vi "initialization.vi"(9 "软件版本":refnum<vi>, 10 "updateconfiguration":refnum<vi>) -> ()   [LabVIEW 2016, in "数据传输系统.lvlib"]
uses:
  <vilib>/Utility/config.llb/Read Key (String).vi
  <vilib>/Utility/config.llb/NI_LVConfig.lvlib
panel:
  in  "参数数值":T1={"CODMn"=TRUE, "CODCr"=TRUE, "DO"=TRUE, "铜"=TRUE, "PH"=TRUE, "氨氮"=TRUE, "比电导率"=TRUE, "水温"=TRUE, "COD"=TRUE, "浊度"=TRUE, "总氮"=TRUE, "总磷"=TRUE, "叶绿素a"=TRUE, "藻密度"=TRUE, "水位"=TRUE, "流速"=TRUE, "瞬时流量"=TRUE, "累积流量"=TRUE, "亚硝氮"=TRUE, "硫化物"=TRUE, "ORP"=TRUE, "铅"=TRUE, "镉"=TRUE, "锌"=TRUE, "镍"=TRUE, "锰"=TRUE, "汞"=TRUE, "气温"=TRUE, "气压"=TRUE, "风速"=TRUE, "风向"=TRUE, "盐度"=TRUE, "磷酸盐"=TRUE, "硝氮"=TRUE, "氟化物"=TRUE, "挥发酚"=TRUE, "氯化物"=TRUE}
  out "配置表格":string[][](table)
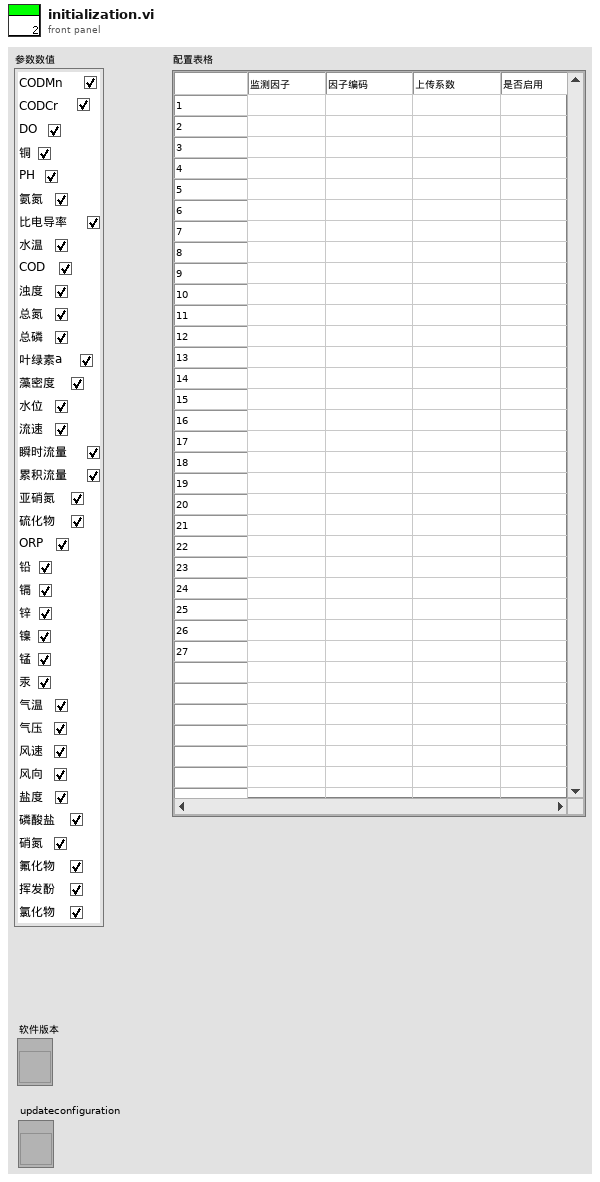
[diagram p1: front panel]
types:
  T1 = cluster{"CODMn":bool, "CODCr":bool, "DO":bool, "铜":bool, "PH":bool, "氨氮":bool, "比电导率":bool, "水温":bool, "COD":bool, "浊度":bool, "总氮":bool, "总磷":bool, "叶绿素a":bool, "藻密度":bool, "水位":bool, "流速":bool, "瞬时流量":bool, "累积流量":bool, "亚硝氮":bool, "硫化物":bool, "ORP":bool, "铅":bool, "镉":bool, "锌":bool, "镍":bool, "锰":bool, "汞":bool, "气温":bool, "气压":bool, "风速":bool, "风向":bool, "盐度":bool, "磷酸盐":bool, "硝氮":bool, "氟化物":bool, "挥发酚":bool, "氯化物":bool}
  T2 = cluster{"setini":string, "sysini":string, "hechaini":string, "actualwrite":string, "actualread":string, "datasent":string, "反控命令信息队列":string, "反控与仪器交互":string}
  T3 = cluster{"主机":string, "用户":string, "密码":string, "远程路径":string, "下载文件名":string, "软件版本":string}
  T4 = cluster{"CODMn":string, "CODCr":string, "DO":string, "铜":string, "PH":string, "氨氮":string, "比电导率":string, "水温":string, "COD":string, "浊度":string, "总氮":string, "总磷":string, "叶绿素a":string, "藻密度":string, "水位":string, "流速":string, "瞬时流量":string, "累积流量":string, "亚硝酸盐":string, "硫化物":string, "ORP":string, "铅":string, "镉":string, "锌":string, "镍":string, "锰":string, "汞":string, "气温":string, "气压":string, "风速":string, "风向":string, "盐度":string, "磷酸盐":string, "硝氮":string, "氟化物":string, "挥发酚":string, "氯化物":string}
  T5 = typedef "NI_LVConfig.lvlib/Config Data RefNum.ctl" = refnum<k1>
  T6 = cluster{"[0]":string, "[1]":string, "[2]":string, "[3]":string, "[4]":string, "[5]":string, "[6]":string, "[7]":string, "[8]":string, "[9]":string, "[10]":string, "[11]":string, "[12]":string, "[13]":string, "[14]":string, "[15]":string, "[16]":string, "[17]":string, "[18]":string, "[19]":string, "[20]":string, "[21]":string, "[22]":string, "[23]":string, "[24]":string, "[25]":string, "[26]":string, "[27]":string, "[28]":string, "[29]":string, "[30]":string, "[31]":string, "[32]":string, "[33]":string, "[34]":string, "[35]":string, "[36]":string}
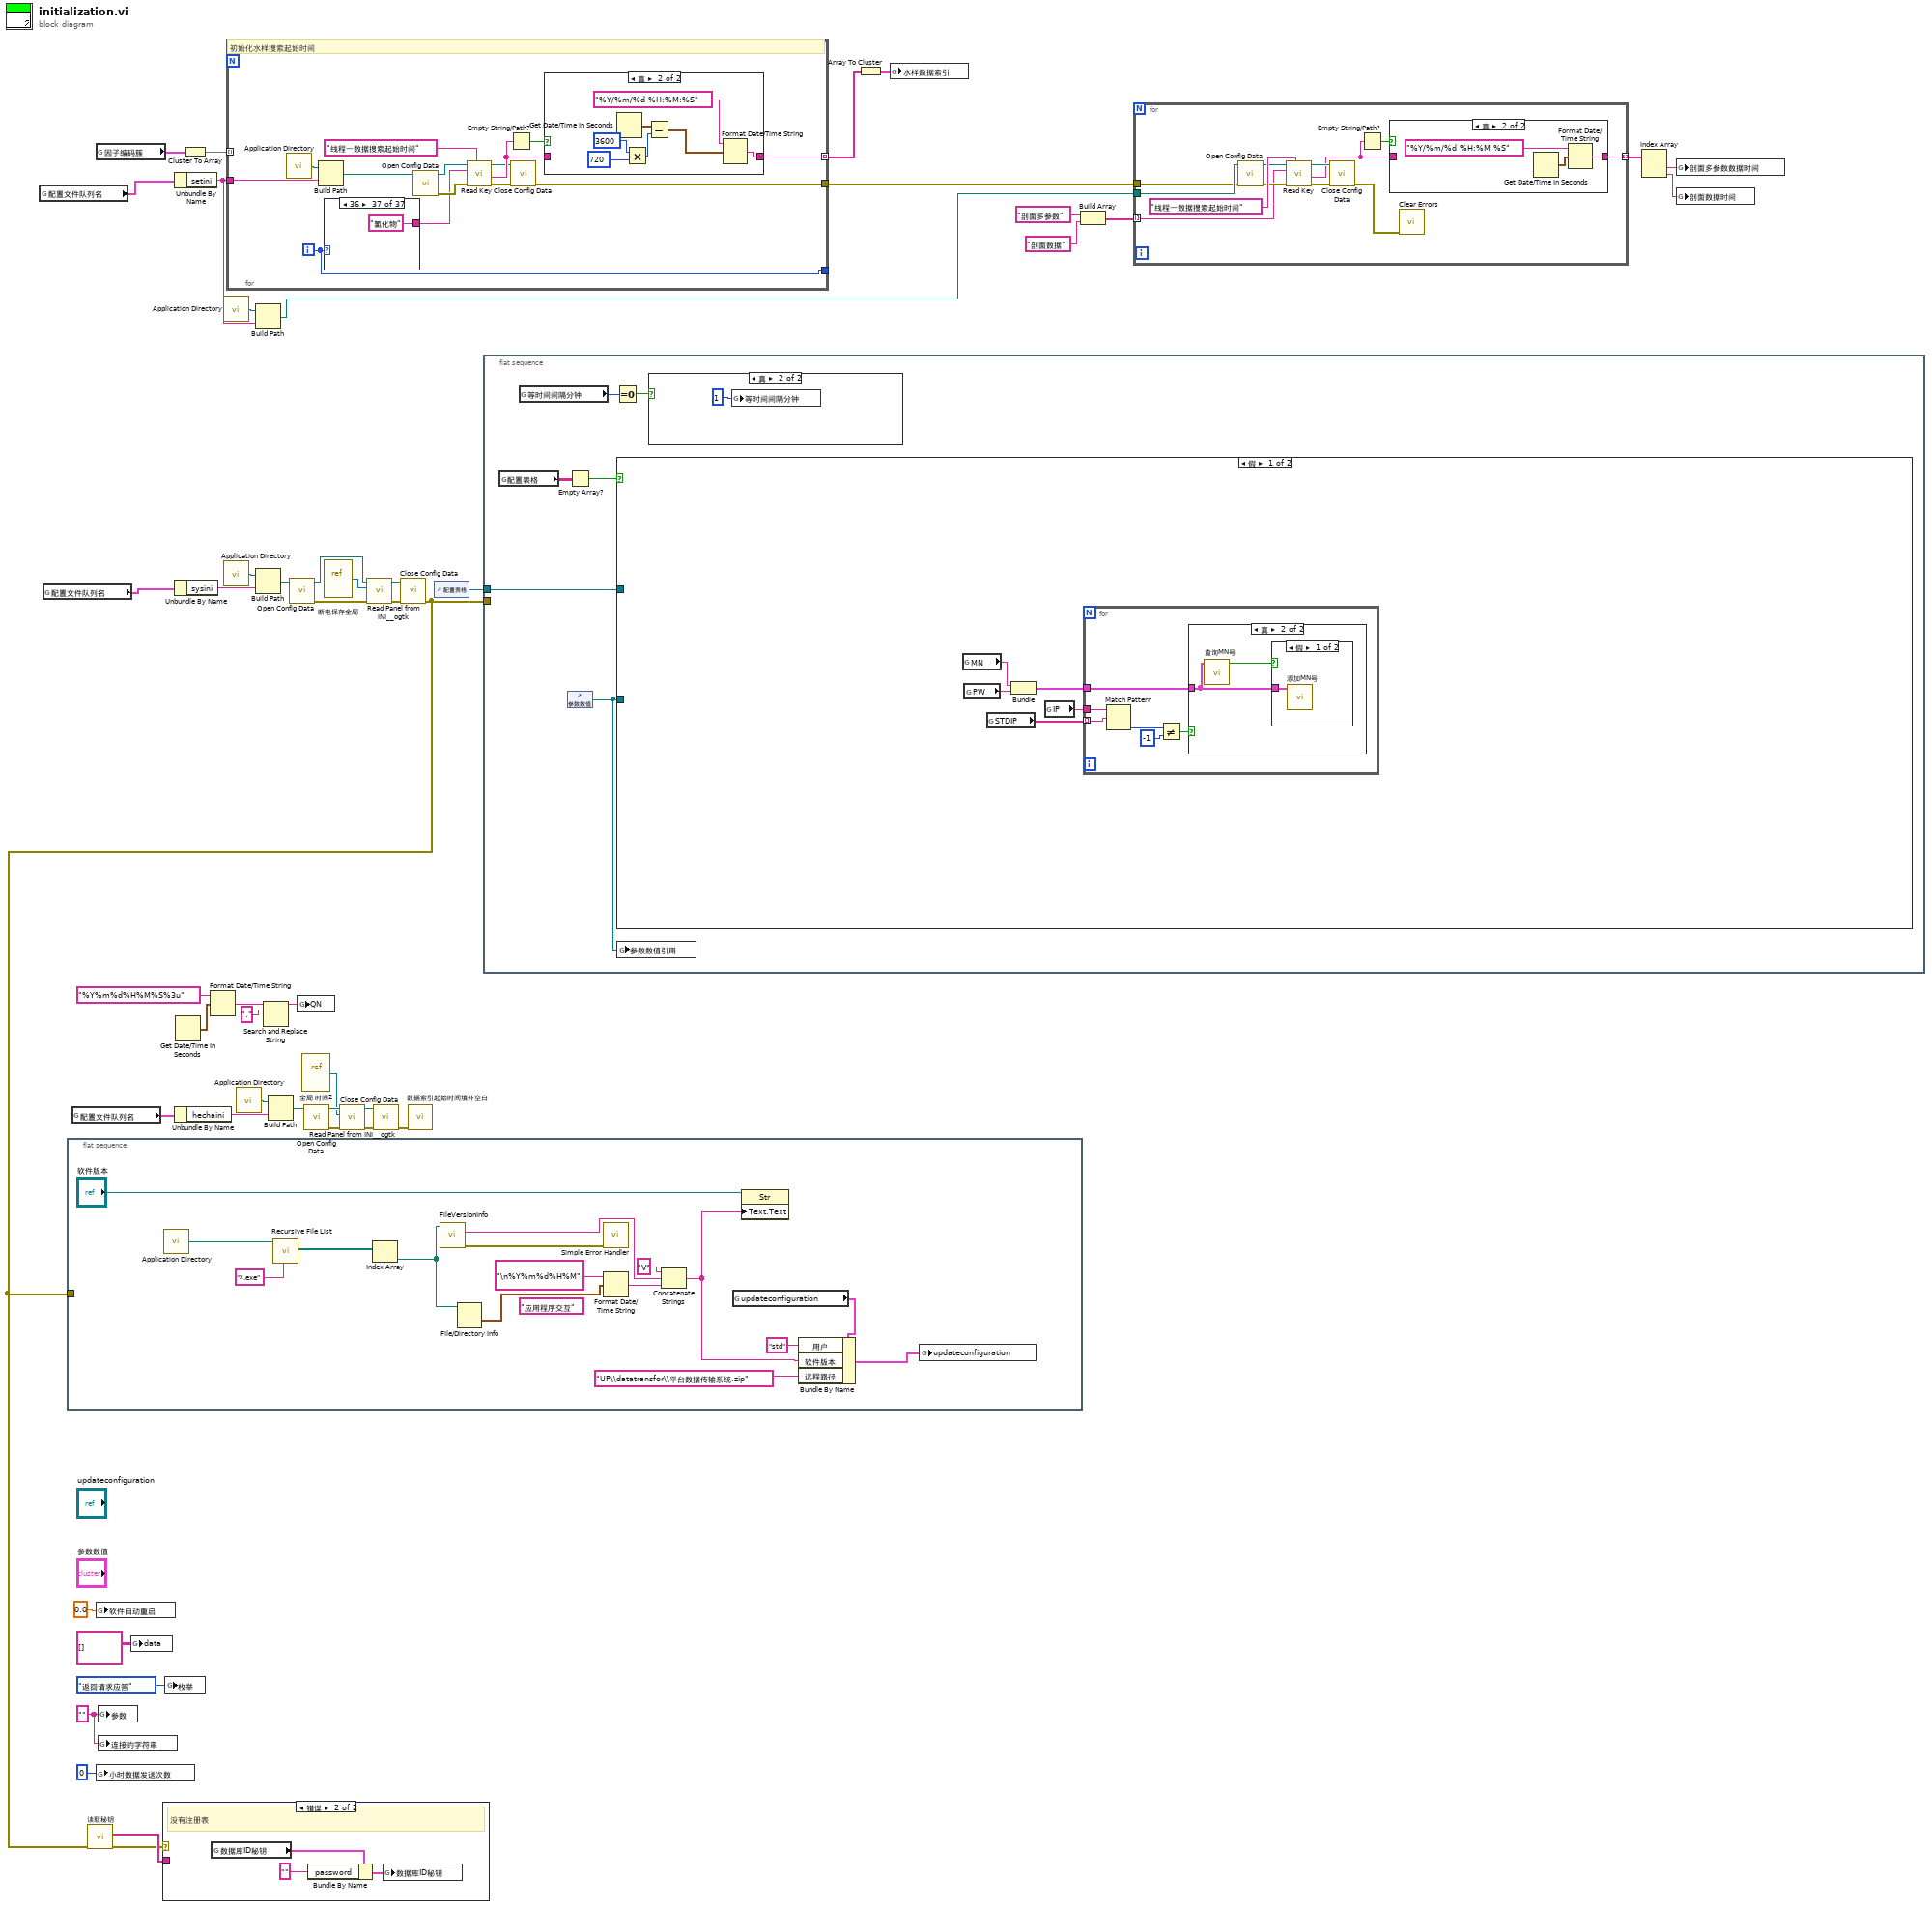
[diagram p0: block diagram]
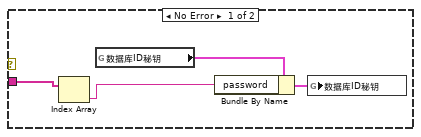
[diagram p2: hidden frame]
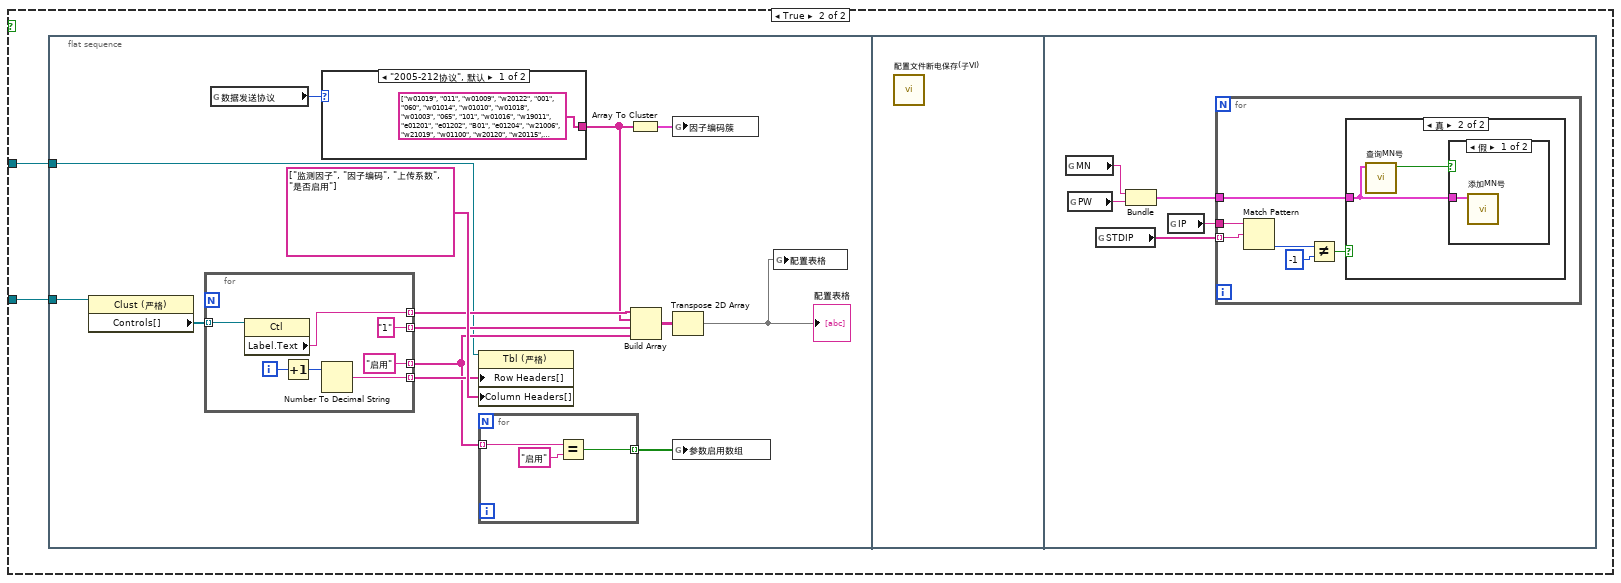
[diagram p6: hidden frame]
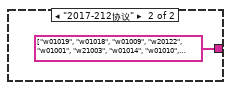
[diagram p7: hidden frame]
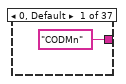
[diagram p12: hidden frame]
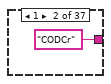
[diagram p13: hidden frame]
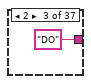
[diagram p14: hidden frame]
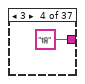
[diagram p15: hidden frame]
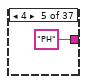
[diagram p16: hidden frame]
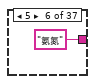
[diagram p17: hidden frame]
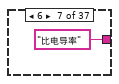
[diagram p18: hidden frame]
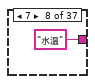
[diagram p19: hidden frame]
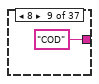
[diagram p20: hidden frame]
diagram:
  w9 = "" ("参数")
  n1 = global read "全局1.vi" "配置文件队列名"() -> (w4:T2)
  n2 = global read "全局1.vi" "配置文件队列名"() -> (w5:T2)
  n3 = flat-sequence {
    tunnel: w2 -> [_]
    frame #0 {
      (unwired) "应用程序交互" ("section")
      n4 = call <vilib>:"Application Directory.vi"() -> ("Application Directory"=w62:path)
      n5 = call <vilib>:"Recursive File List.vi"("pattern"="*.exe", "Folder Path"=w62) -> ("All Files in Dir"=w56:path[])  [unwired: 5 in, 4 out]
      n6 = Index Array(array=w56) -> (element=w57:path)  [unwired: 1 in]
      n7 = call <vilib>:"FileVersionInfo.vi"("Application Path in"=w57) -> ("error out"=w63:errorcluster, "File Version Info"=w64:string)  [unwired: 7 in, 2 out]
      n8 = File/Directory Info(path=w57) -> (last mod=w58:timestamp)  [unwired: 1 in, 6 out]
      n9 = call <vilib>:"Simple Error Handler.vi"("error in (no error)"=w63) -> ()  [unwired: 4 in, 5 out]
      n10 = Format Date/Time String(time format string (%c)="\n%Y%m%d%H%M" ("时间格式字符串(%c)"), seconds (now)=w58) -> (date/time string=w61:string)  [unwired: 1 in]
      n11 = Concatenate Strings("V" ("字符串"), w64, w61) -> (w53:string)
      n12 = global read "断电保存全局.vi" "updateconfiguration"() -> (w50:T3)
      n13 = property class="Str"(reference="软件版本", "Text.Text"=w53) -> ()  [unwired: 1 in, 2 out]
      n14 = Bundle By Name(cluster=w50, "用户"="std", "软件版本"=w53, "远程路径"="UP\\datatransfor\\平台数据传输系统.zip") -> (w52:T3)
      n15 = global write "断电保存全局.vi" "updateconfiguration"(w52) -> ()
    }
  }
  n16 = global read "全局1.vi" "配置文件队列名"() -> (w6:T2)
  n17 = global read "断电保存全局.vi" "因子编码簇"() -> (w38:T4)
  n18 = global write "全局1.vi" "软件自动重启"(0.0 ("软件自动重启")) -> ()
  n19 = global write "全局 小时数据发送次数.vi" "小时数据发送次数"(0 ("数值")) -> ()
  n20 = global write "全局 实时数据参数.vi" "参数"(w9) -> ()
  n21 = global write "全局 实时数据参数.vi" "连接的字符串"(w9) -> ()
  n22 = global write "全局 实时数据参数.vi" "data"(string[][] [] ("data")) -> ()
  n23 = global write "全局1.vi" "枚举"(enum16{"返回请求应答", "上传数据", "返回执行结果"}."返回请求应答" ("枚举")) -> ()
  n24 = Unbundle By Name(w4) -> ("setini"=w40:string)
  n25 = Unbundle By Name(w5) -> ("sysini"=w41:string)
  n26 = Unbundle By Name(w6) -> ("hechaini"=w42:string)
  n27 = Get Date/Time In Seconds() -> (seconds since 1Jan1904=w13:timestamp)
  n28 = Cluster To Array(cluster=w38) -> (array=w32:string[])
  n29 = Format Date/Time String(time format string (%c)="%Y%m%d%H%M%S%3u" ("时间格式字符串(%c)"), seconds (now)=w13) -> (date/time string=w14:string)  [unwired: 1 in]
  n30 = call <vilib>:"Application Directory.vi"() -> ("Application Directory"=w35:path)
  n31 = call <vilib>:"Application Directory.vi"() -> ("Application Directory"=w21:path)
  n32 = for {
    tunnel: w32 -> [_] mode=indexing
    tunnel: [w70] -> _
    tunnel: [w67] -> w33 mode=indexing
    tunnel: [w66] -> w37
    tunnel: w40 -> [w65]
    i -> [w70]
    # "初始化水样搜索起始时间"
    n33 = call <vilib>:"Application Directory.vi"() -> ("Application Directory"=w78:path)
    n34 = Build Path(base path=w78, name or relative path=w65) -> (appended path=w77:path)
    n35 = case shown="36" w70 {
      tunnel: ["CODMn" "CODCr" "DO" "铜" "PH" "氨氮" "比电导率" "水温" "COD" "浊度" "总氮" "总磷" "叶绿素a" "藻密度" "水位" "流速" "瞬时流量" "累积流量" "亚硝氮" "硫化物" "ORP" "铅" "镉" "锌" "镍" "锰" "汞" "气温" "气压" "风速" "风向" "盐度" "磷酸盐" "硝氮" "氟化物" "挥发酚" "氯化物"] -> w73
      frame 0, Default {
      }
      frame 1 {
      }
      frame 2 {
      }
      frame 3 {
      }
      frame 4 {
      }
      frame 5 {
      }
      frame 6 {
      }
      frame 7 {
      }
      frame 8 {
      }
      frame 9 {
      }
      frame 10 {
      }
      frame 11 {
      }
      frame 12 {
      }
      frame 13 {
      }
      frame 14 {
      }
      frame 15 {
      }
      frame 16 {
      }
      frame 17 {
      }
      frame 18 {
      }
      frame 19 {
      }
      frame 20 {
      }
      frame 21 {
      }
      frame 22 {
      }
      frame 23 {
      }
      frame 24 {
      }
      frame 25 {
      }
      frame 26 {
      }
      frame 27 {
      }
      frame 28 {
      }
      frame 29 {
      }
      frame 30 {
      }
      frame 31 {
      }
      frame 32 {
      }
      frame 33 {
      }
      frame 34 {
      }
      frame 35 {
      }
      frame 36 {
      }
    }
    n36 = call <vilib>:"Open Config Data.vi"("configuration file path"=w77) -> ("error out"=w75:errorcluster, "refnum"=w76:T5)  [unwired: 8 in, 1 out]
    n37 = call-poly <vilib>:"Read Key.vi"("section"="线程一数据搜索起始时间", "error in (no error)"=w75, "key"=w73, "refnum"=w76) -> ("error out"=w68:errorcluster, "value"=w71:string, "refnum out"=w69:T5)  [unwired: 4 in, 1 out]
    n38 = Empty String/Path?(string/path=w71) -> (empty?=w72:bool)
    n39 = call <vilib>:"Close Config Data.vi"("error in (no error)"=w68, "refnum"=w69) -> ("error out"=w66:errorcluster)  [unwired: 8 in, 1 out]
    n40 = case shown="真" w72 {
      tunnel: [w79 w85] -> w67
      tunnel: w71 -> [w79 _]
      frame False {
      }
      frame True {
        n41 = Get Date/Time In Seconds() -> (seconds since 1Jan1904=w84:timestamp)
        n42 = Multiply(x=3600, y=720) -> (x*y=w81:i32)
        n43 = Subtract(x=w84, y=w81) -> (x-y=w80:timestamp)
        n44 = Format Date/Time String(time format string (%c)="%Y/%m/%d %H:%M:%S" ("时间格式字符串(%c)"), seconds (now)=w80) -> (date/time string=w85:string)  [unwired: 1 in]
      }
    }
  }
  n45 = call <vilib>:"Application Directory.vi"() -> ("Application Directory"=w25:path)
  n46 = Build Path(base path=w35, name or relative path=w40) -> (appended path=w36:path)
  n47 = Build Path(base path=w21, name or relative path=w41) -> (appended path=w22:path)
  n48 = Search and Replace String(input string=w14, search string="." ("搜索字符串")) -> (result string=w16:string)  [unwired: 6 in, 3 out]
  n49 = Build Path(base path=w25, name or relative path=w42) -> (appended path=w24:path)
  n50 = call <vilib>:"Open Config Data.vi"("configuration file path"=w22) -> ("error out"=w17:errorcluster, "refnum"=w18:T5)  [unwired: 8 in, 1 out]
  n51 = global write "全局1.vi" "QN"(w16) -> ()
  n52 = vi-ref "全局 时间2.vi"() -> (w27:refnum<vi>)
  n53 = call <vilib>:"Open Config Data.vi"("configuration file path"=w24) -> ("error out"=w29:errorcluster, "refnum"=w28:T5)  [unwired: 8 in, 1 out]
  n54 = vi-ref "断电保存全局.vi"() -> (w19:refnum<vi>)
  n55 = call <userlib>:"Read Panel from INI__ogtk.vi"("error in (no error)"=w29, "VI ref"=w27, "refnum"=w28) -> ("error out"=w30:errorcluster, "refnum out"=w26:T5)  [unwired: 7 in]
  n56 = call <userlib>:"Read Panel from INI__ogtk.vi"("error in (no error)"=w17, "VI ref"=w19, "refnum"=w18) -> ("error out"=w23:errorcluster, "refnum out"=w20:T5)  [unwired: 7 in]
  n57 = call <vilib>:"Close Config Data.vi"("error in (no error)"=w30, "refnum"=w26) -> ("error out"=w31:errorcluster)  [unwired: 8 in, 1 out]
  n58 = call <vilib>:"Close Config Data.vi"("error in (no error)"=w23, "refnum"=w20) -> ("error out"=w2:errorcluster)  [unwired: 8 in, 1 out]
  n59 = call "读取秘钥.vi"("error in (no error)"=w2) -> ("error out"=w1:errorcluster, "值"=w3:string[])  [unwired: 8 in, 1 out]
  n60 = case shown="错误" w1 {
    tunnel: w3 -> [w127 _]
    frame No Error {
      n61 = Index Array(array=w127) -> (element=w124:string)  [unwired: 1 in]
      n62 = global read "外部交互全局.vi" "数据库ID秘钥"() -> (w125:cluster{"userID":string, "password":string})
      n63 = Bundle By Name(cluster=w125, "password"=w124) -> (w126:cluster{"userID":string, "password":string})
      n64 = global write "外部交互全局.vi" "数据库ID秘钥"(w126) -> ()
    }
    frame Error {
      # "没有注册表"
      n65 = global read "外部交互全局.vi" "数据库ID秘钥"() -> (w128:cluster{"userID":string, "password":string})
      n66 = Bundle By Name(cluster=w128, "password"="") -> (w129:cluster{"userID":string, "password":string})
      n67 = global write "外部交互全局.vi" "数据库ID秘钥"(w129) -> ()
    }
  }
  n68 = call "数据索引起始时间填补空白.vi"("error in (no error)"=w31) -> ()  [unwired: 10 in, 1 out]
  n69 = control-ref of="配置表格"() -> (w7:refnum<vi>)
  n70 = flat-sequence {
    tunnel: w2 -> [_]
    tunnel: w7 -> [w134]
    frame #0 {
      n71 = global read "断电保存全局.vi" "配置表格"() -> (w136:string[][])
      n72 = global read "断电保存全局.vi" "等时间间隔分钟"() -> (w131:i32)
      n73 = Empty Array?(array=w136) -> (empty?=w135:bool)
      n74 = control-ref of="参数数值"() -> (w133:refnum<vi>)
      n75 = Equal To 0?(x=w131) -> (x = 0?=w132:bool)
      n76 = case shown="假" w135 {
        tunnel: w134 -> [_ w153]
        tunnel: w133 -> [_ w152]
        frame False {
          n77 = global read "断电保存全局.vi" "MN"() -> (w142:string)
          n78 = global read "断电保存全局.vi" "PW"() -> (w141:string)
          n79 = global read "断电保存全局.vi" "STDIP"() -> (w139:string[])
          n80 = Bundle("MN"=w142, "PW"=w141) -> (w140:cluster{"MN":string, "PW":string})  [unwired: 1 in]
          n81 = global read "断电保存全局.vi" "IP"() -> (w138:string)
          n82 = for {
            tunnel: w139 -> [w148] mode=indexing
            tunnel: w138 -> [w147]
            tunnel: w140 -> [w143]
            n83 = Match Pattern(string=w147, regular expression=w148) -> (offset past match=w146:i32)  [unwired: 1 in, 3 out]
            n84 = Not Equal?(x=w146, y=-1) -> (x != y?=w144:bool)
            n85 = case shown="真" w144 {
              tunnel: w143 -> [_ w150]
              frame False {
              }
              frame True {
                n86 = call "查询MN号.vi"("簇"=w150) -> ("包含启动项"=w149:bool)  [unwired: 9 in, 1 out]
                n87 = case shown="假" w149 {
                  tunnel: w150 -> [w151 _]
                  frame False {
                    n88 = call "添加MN号.vi"("簇"=w151) -> ()  [unwired: 9 in, 2 out]
                  }
                  frame True {
                  }
                }
              }
            }
          }
        }
        frame True {
          n89 = flat-sequence {
            tunnel: w153 -> [w155]
            tunnel: w152 -> [w154]
            frame #0 {
              n90 = property on="属性节点" class="Clust (严格)"(reference=w154) -> ("Controls[]"=w163:refnum<vi>[])  [unwired: 1 in, 2 out]
              n91 = for {
                tunnel: w163 -> [w179] mode=indexing
                tunnel: [w178] -> w165 mode=indexing
                tunnel: [w176] -> w164 mode=indexing
                tunnel: ["1"] -> w158 mode=indexing
                tunnel: ["启用"] -> w157 mode=indexing
                i -> [w177]
                n92 = property class="Ctl"(reference=w179) -> ("Label.Text"=w178:string)  [unwired: 1 in, 2 out]
                n93 = Increment(x=w177) -> (x+1=w175:i32)
                n94 = Number To Decimal String(number=w175) -> (decimal integer string=w176:string)  [unwired: 1 in]
              }
              n95 = global read "断电保存全局.vi" "数据发送协议"() -> (w161:enum16{"2005-212协议", "2017-212协议"})
              n96 = case shown="\"2005-212协议\", 默认" w161 {
                tunnel: [string[] ["w01019", "011", "w01009", "w20122", "001", "060", "w01014", "w01010", "w01018", "w01003", "065", "101", "w01016", "w19011", "e01201", "e01202", "B01", "e01204", "w21006", "w21019", "w01100", "w20120", "w20115", "w20123", "w20121", "w20124", "w20111", "a01001", "a01006", "a01007", "a01008", "w01002", "w21015", "w21007", "w21017", "w23002", "w21002"] string[] ["w01019", "w01018", "w01009", "w20122", "w01001", "w21003", "w01014", "w01010", "w01018", "w01003", "w21001", "w21011", "w01016", "w19011", "e01201", "e01202", "e01203", "e01204", "w21006", "w21019", "w01100", "w20120", "w20115", "w20123", "w20121", "w20124", "w20111", "a01001", "a01006", "a01007", "a01008", "w01002", "w21015", "w21007", "w21017", "w23002", "w21002"]] -> w159
                frame "2005-212协议", Default {
                }
                frame "2017-212协议" {
                }
              }
              n97 = property on="属性节点" class="Tbl (严格)"(reference=w155, "Row Headers[]"=w164, "Column Headers[]"=string[] ["监测因子", "因子编码", "上传系数", "是否启用"]) -> ()  [unwired: 1 in, 2 out]
              n98 = for {
                tunnel: w157 -> [w170] mode=indexing
                tunnel: [w168] -> w156 mode=indexing
                n99 = Equal?(x=w170, y="启用") -> (x = y?=w168:bool)
              }
              n100 = Array To Cluster(array=w159) -> (cluster=w160:T6)
              n101 = Build Array(w165, w159, w158, w157) -> (w167:string[][])
              n102 = global write "断电保存全局.vi" "因子编码簇"(w160) -> ()
              n103 = Transpose 2D Array(2D array=w167) -> (transposed array=w162:string[][])
              "配置表格" <- w162
              n104 = global write "断电保存全局.vi" "参数启用数组"(w156) -> ()
              n105 = global write "断电保存全局.vi" "配置表格"(w162) -> ()
            }
            frame #1 {
              n106 = call "配置文件断电保存(子VI).vi"() -> ()  [unwired: 12 in]
            }
            frame #2 {
              n107 = global read "断电保存全局.vi" "MN"() -> (w184:string)
              n108 = global read "断电保存全局.vi" "PW"() -> (w183:string)
              n109 = global read "断电保存全局.vi" "STDIP"() -> (w181:string[])
              n110 = Bundle("MN"=w184, "PW"=w183) -> (w182:cluster{"MN":string, "PW":string})  [unwired: 1 in]
              n111 = global read "断电保存全局.vi" "IP"() -> (w180:string)
              n112 = for {
                tunnel: w181 -> [w190] mode=indexing
                tunnel: w180 -> [w189]
                tunnel: w182 -> [w185]
                n113 = Match Pattern(string=w189, regular expression=w190) -> (offset past match=w188:i32)  [unwired: 1 in, 3 out]
                n114 = Not Equal?(x=w188, y=-1) -> (x != y?=w186:bool)
                n115 = case shown="真" w186 {
                  tunnel: w185 -> [_ w192]
                  frame False {
                  }
                  frame True {
                    n116 = call "查询MN号.vi"("簇"=w192) -> ("包含启动项"=w191:bool)  [unwired: 9 in, 1 out]
                    n117 = case shown="假" w191 {
                      tunnel: w192 -> [w193 _]
                      frame False {
                        n118 = call "添加MN号.vi"("簇"=w193) -> ()  [unwired: 9 in, 2 out]
                      }
                      frame True {
                      }
                    }
                  }
                }
              }
            }
          }
        }
      }
      n119 = global write "断电保存全局.vi" "参数数值引用"(w133) -> ()
      n120 = case shown="真" w132 {
        frame False {
        }
        frame True {
          n121 = global write "断电保存全局.vi" "等时间间隔分钟"(1 ("等时间间隔分钟")) -> ()
        }
      }
    }
  }
  n122 = Array To Cluster(array=w33) -> (cluster=w34:T6)
  n123 = global write "全局 水样时间.vi" "水样数据索引"(w34) -> ()
  n124 = Build Array("剖面多参数" ("key"), "剖面数据" ("key")) -> (w45:string[])
  n125 = for {
    tunnel: w36 -> [w205]
    tunnel: w37 -> [w204]
    tunnel: w45 -> [w196] mode=indexing
    tunnel: [w195] -> w46 mode=indexing
    n126 = call <vilib>:"Open Config Data.vi"("error in (no error)"=w204, "configuration file path"=w205) -> ("error out"=w201:errorcluster, "refnum"=w202:T5)  [unwired: 7 in, 1 out]
    n127 = call-poly <vilib>:"Read Key.vi"("section"="线程一数据搜索起始时间", "error in (no error)"=w201, "key"=w196, "refnum"=w202) -> ("error out"=w199:errorcluster, "value"=w198:string, "refnum out"=w200:T5)  [unwired: 4 in, 1 out]
    n128 = call <vilib>:"Close Config Data.vi"("error in (no error)"=w199, "refnum"=w200) -> ("error out"=w194:errorcluster)  [unwired: 8 in, 1 out]
    n129 = Empty String/Path?(string/path=w198) -> (empty?=w197:bool)
    n130 = case shown="真" w197 {
      tunnel: [w206 w207] -> w195
      tunnel: w198 -> [w206 _]
      frame False {
      }
      frame True {
        n131 = Get Date/Time In Seconds() -> (seconds since 1Jan1904=w209:timestamp)
        n132 = Format Date/Time String(time format string (%c)="%Y/%m/%d %H:%M:%S" ("时间格式字符串(%c)"), seconds (now)=w209) -> (date/time string=w207:string)  [unwired: 1 in]
      }
    }
    n133 = call <vilib>:"Clear Errors.vi"("error in (no error)"=w194) -> ()  [unwired: 5 in, 2 out]
  }
  n134 = Index Array(array=w46) -> (element #1=w47:string, element #2=w48:string)  [unwired: 2 in]
  n135 = global write "全局 水样时间.vi" "剖面多参数数据时间"(w47) -> ()
  n136 = global write "全局 水样时间.vi" "剖面数据时间"(w48) -> ()
